vi "Wait for Axis Arrival at Target Position.vi"(4 "error in (no error)":errorcluster, 6 "Axis In":i16, 7 "Controller Reference":refnum<k7>) -> (0 "error out":errorcluster, 1 "Axis not moving":bool, 2 "Axis Out":i16, 3 "Controller Reference out":refnum<k7>)   [LabVIEW 2015]
doc: "Waits for the input Axis to arrive at it's set Target Position. Can detect if the Axis is not moving towards it's target position and outputs a Boolean to indicate this."
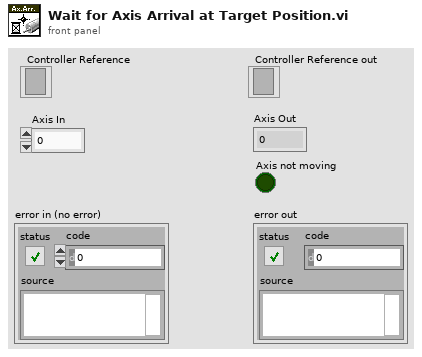
[diagram p1: front panel]
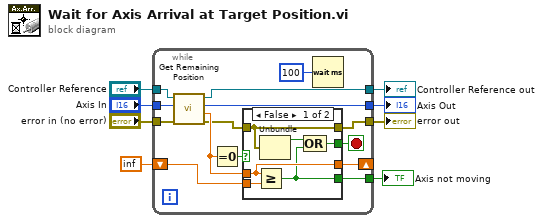
[diagram p0: block diagram]
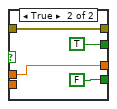
[diagram p2: hidden frame]
diagram:
  n1 = while {
    tunnel: "Axis In" -> [w22]
    tunnel: "Controller Reference" -> [w21]
    tunnel: [w20] -> w6
    tunnel: [w19] -> w5
    shift-right: [w11] -> _
    shift-left: sgl inf -> [w15]
    tunnel: "error in (no error)" -> [w18]
    tunnel: [w13] -> w2
    tunnel: [w10] -> w1
    stop <- w16 stop-if-true
    n2 = call "Get Remaining Position.vi"("error in (no error)"=w18, "Axis In"=w22, "Controller Reference"=w21) -> ("error out"=w12:errorcluster, "Position Remaining"=w14:sgl, "Axis Out"=w19:i16, "Controller Reference out"=w20:refnum<k7>)  [unwired: 1 in]
    n3 = Equal To 0?(x=w14) -> (x = 0?=w17:bool)
    n4 = case shown="False" w17 {
      tunnel: [w25 TRUE] -> w16
      tunnel: w15 -> [w28 _]
      tunnel: w14 -> [w26 w30]
      tunnel: [w24 w31] -> w13
      tunnel: w12 -> [w24 w31]
      tunnel: [w26 w30] -> w11
      tunnel: [w23 FALSE] -> w10
      frame False {
        n5 = Greater Or Equal?(x=w26, y=w28) -> (x >= y?=w23:bool)
        n6 = Unbundle(w24) -> ("status"=w27:bool)  [unwired: 2 out]
        n7 = Compound Arithmetic op=OR(w27, w23) -> (w25:bool)
      }
      frame True {
      }
    }
    n8 = Wait (ms)(milliseconds to wait=u32 100) -> ()  [unwired: 1 out]
  }
  "Controller Reference out" <- w6
  "Axis Out" <- w5
  "error out" <- w2
  "Axis not moving" <- w1
